vi "VI Server_Get Menu Ring Selection_FromReference.vi"(7 "Menu-Ring.Ref":refnum<vi>, 8 "error in":errorcluster, 11 "VI Server Cluster":T1) -> (0 "error out":errorcluster, 1 "Control Reference":refnum<vi>, 2 "Selection":string, 3 "VI Server Custer.DUP":T1={"VI Ref"=refnum, "Refs"=[], "Labels"=["Label", "Size", "Font", "Heght", "Width", "Ledding Denominator", "Ledding Nominator", "Label Number", "Microstep Resolution", "X", "Y", "Z", "Italic?", "Underlined?"]}, 4 "Value":u16, 6 "Label.Text":string)   [LabVIEW 2020]
doc: "Returns Item Name selected of the Text Ring."
uses:
  VI Server Toolkit LV2013.lvlib
  VI Server Cluster.ctl
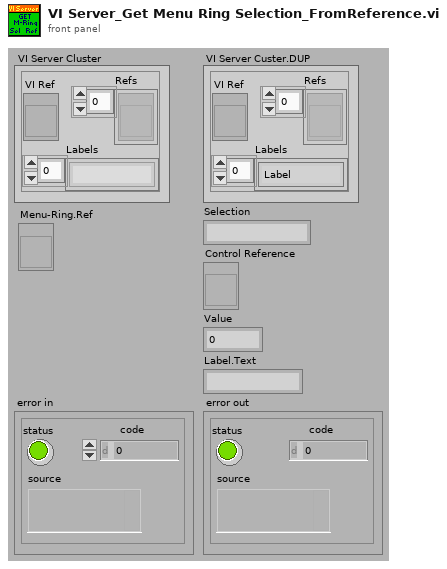
[diagram p1: front panel]
types:
  T1 = typedef "VI Server Toolkit LV2013.lvlib/VI Server Cluster.ctl" = cluster{"VI Ref":refnum<vi>, "Refs":refnum<vi>[], "Labels":string[]}
  T2 = typedef "LVStringsAndValuesArrayTypeDef_U16.ctl" = cluster{"String":string, "Value":u16}[]
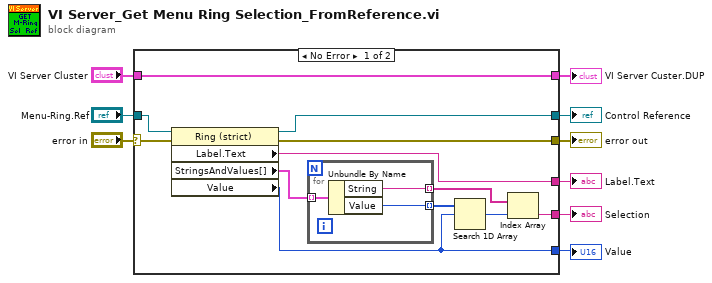
[diagram p0: block diagram]
diagram:
  n1 = case shown="No Error" "error in" {
    selector: "error in" -> [w21 w25]
    tunnel: "VI Server Cluster" -> [w18 _]
    tunnel: [w20 w25] -> w9
    tunnel: [w10 _] -> w6
    tunnel: [w13 _] -> w5
    tunnel: [w12 _] -> w4
    tunnel: [w19 _] -> w3
    tunnel: [w18 _] -> w2
    tunnel: "Menu-Ring.Ref" -> [w11 _]
    frame No Error {
      n2 = property class="Ring (strict)"(reference=w11, error in=w21) -> (reference out=w10:refnum<vi>, error out=w20:errorcluster, "Label.Text"=w19:string, "StringsAndValues[]"=w17:T2, "Value"=w12:u16)
      n3 = for {
        tunnel: w17 -> [w24] mode=indexing
        tunnel: [w23] -> w16 mode=indexing
        tunnel: [w22] -> w14 mode=indexing
        n4 = Unbundle By Name(w24) -> ("String"=w22:string, "Value"=w23:u16)
      }
      n5 = Search 1D Array(1D array=w16, element=w12) -> (index of element=w15:i32)  [unwired: 1 in]
      n6 = Index Array(array=w14, index=w15) -> (element=w13:string)
    }
    frame Error {
      n7 = call "VI Server_Empty VI Server Cluster.vi"() -> ()  [unwired: 7 in, 1 out]
    }
  }
  "error out" <- w9
  "VI Server Custer.DUP" <- w2
  "Control Reference" <- w6
  "Selection" <- w5
  "Value" <- w4
  "Label.Text" <- w3
